vi "Handle error.vi"(8 "error in (no error)":T2, 10 "module loopdata":T3, 11 "state in":T1) -> (3 "state out":T1)   [LabVIEW 2019, in "Communication Interface.lvlib"]
uses:
  Communication Interface.lvlib
  module data.ctl
  Intertarget communication/CR_master_class/CR_master.lvclass
  Intertarget communication/CR slave_class/CR slave.lvclass
  module state.ctl
  SubVIs/Shared/Shared.lvlib
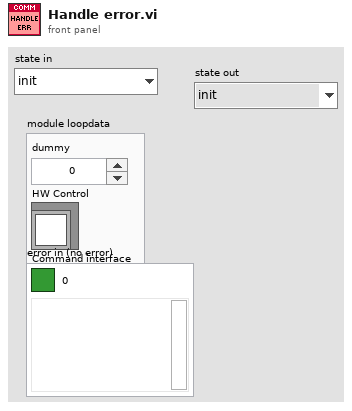
[diagram p1: front panel]
types:
  T1 = typedef "Communication Interface.lvlib/module state.ctl" = enum16{"init", "wait on connection", "communication", "close"}
  T2 = cluster{"Boolean Round":bool, "code":i32, "source":string}
  T3 = typedef "Communication Interface.lvlib/module data.ctl" = cluster{"dummy":dbl, "HW Control":refnum<class "CR_master.lvclass">, "Command interface":refnum<class "CR slave.lvclass">}
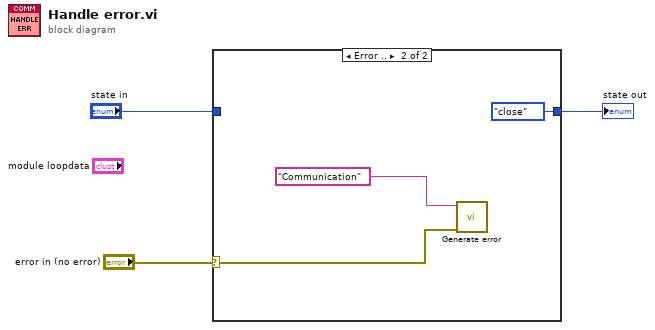
[diagram p0: block diagram]
diagram:
  n1 = case shown="Error .." "error in (no error)" {
    selector: "error in (no error)" -> [_ w6]
    tunnel: [w4 module_state."close" ("state in")] -> w2
    tunnel: "state in" -> [w4 _]
    frame No Error {
    }
    frame Error {
      n2 = call "Generate error.vi"("error in (no error)"=w6, "module"="Communication") -> ()  [unwired: 9 in, 1 out]
    }
  }
  "state out" <- w2
